vi "Scanning Volts to Microns.vi"() -> (0 "Scanning Conversions OUT":T1)   [LabVIEW 2016]
uses:
  Scanning Conversions.ctl
panel:
  in  "Scanning Conversions IN":T1
  # "Copyright (C) 2020 Edward S Allgeyer\n\nRedistribution and use in source and binary forms, with or without\nmodification, are permitted provided that the following conditions\nare met:\n\n1. Redistributions of source code must retain the above copyright\n   notice, this list of conditions and the following disclaimer.\n\n2. Redistributions in binary form must reproduce the above copyright\n   notice, this list of conditions and the following disclaimer in\n   the documentation and/or other materials provided with the\n   distribution.\n\n3. Neither the name of the copyright holder nor the names of its\n   contributors may be used to endorse or promote products derived\n   from this software without specific prior written permission.\n\nTHIS SOFTWARE IS PROVIDED BY THE COPYRIGHT HOLDERS AND CONTRIBUTORS\n\"AS IS\" AND ANY EXPRESS OR IMPLIED WARRANTIES, INCLUDING, BUT NOT\nLIMITED TO, THE IMPLIED WARRANTIES OF MERCHANTABILITY AND FITNESS\nFOR A PARTICULAR PURPOSE ARE DISCLAIMED. IN NO EVENT SHALL THE\nCOPYRIGHT HOLDER OR CONTRIBUTORS BE LIABLE FOR ANY DIRECT, INDIRECT,\nINCIDENTAL, SPECIAL, EXEMPLARY, OR CONSEQUENTIAL DAMAGES (INCLUDING,\nBUT NOT LIMITED TO, PROCUREMENT OF SUBSTITUTE GOODS OR SERVICES;\nLOSS OF USE, DATA, OR PROFITS; OR BUSINESS INTERRUPTION) HOWEVER\nCAUSED AND ON ANY THEORY OF LIABILITY, WHETHER IN CONTRACT, STRICT\nLIABILITY, OR TORT (INCLUDING NEGLIGENCE OR OTHERWISE) ARISING IN\nANY WAY OUT OF THE USE OF THIS SOFTWARE, EVEN IF ADVISED OF THE\nPOSSIBILITY OF SUCH DAMAGE."
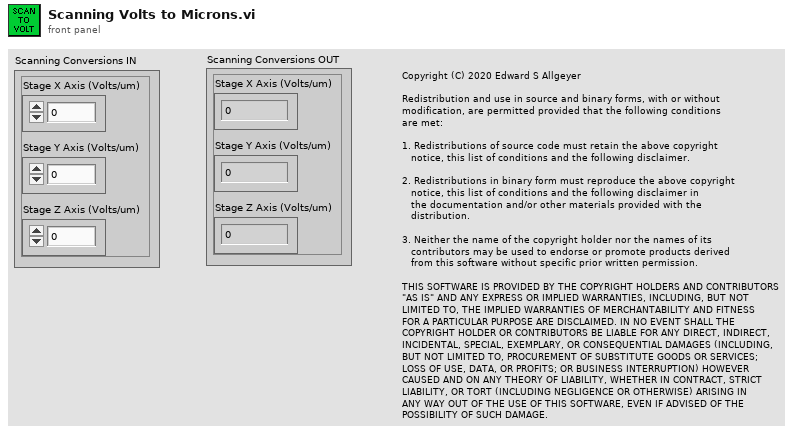
[diagram p1: front panel]
types:
  T1 = typedef "Scanning Conversions.ctl" = cluster{"Stage X Axis (Volts/um)":dbl, "Stage Y Axis (Volts/um)":dbl, "Stage Z Axis (Volts/um)":dbl}
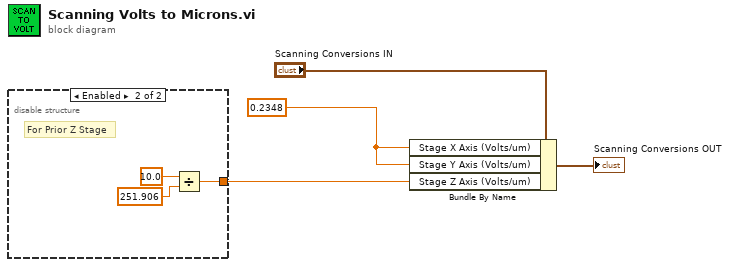
[diagram p0: block diagram]
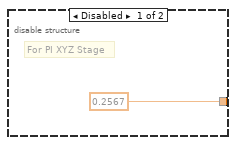
[diagram p2: hidden frame]
diagram:
  w2 = 0.2348
  n1 = disable-structure shown="Enabled" {
    disable-tunnel: [0.2567 ("Stage Z Axis (Volts/um)") w6] -> w1
    frame Disabled {
      # "For PI XYZ Stage"
    }
    frame Enabled {
      # "For Prior Z Stage"
      n2 = Divide(x=10.0, y=251.906) -> (x/y=w6:dbl)
    }
  }
  n3 = Bundle By Name(cluster="Scanning Conversions IN", "Stage X Axis (Volts/um)"=w2, "Stage Y Axis (Volts/um)"=w2, "Stage Z Axis (Volts/um)"=w1) -> (→"Scanning Conversions OUT":T1)
